vi "MainSockets.vi"() -> ()   [LabVIEW 2018]
uses:
  <vilib>/addons/zeromq/zmq_context.lvclass
  socket REP/socket REP.lvclass
  C:/Users/Denis/Desktop/communication-manager/communication-manager/Socket/Socket.lvclass
  socket REQ/socket REQ.lvclass
  socket SUB/socket SUB.lvclass
  socket PUB/socket PUB.lvclass
  RxTx/CM_RxTx.lvclass
  Socket/Socket.lvclass
panel:
  in  "socket PUB.lvclass":refnum<class "socket PUB.lvclass">
  in  "socket SUB.lvclass":refnum<class "socket SUB.lvclass">
  in  "socket REQ.lvclass":refnum<class "socket REQ.lvclass">
  in  "socket REP.lvclass":refnum<class "socket REP.lvclass">
  out "context":refnum<class "zmq_context.lvclass">
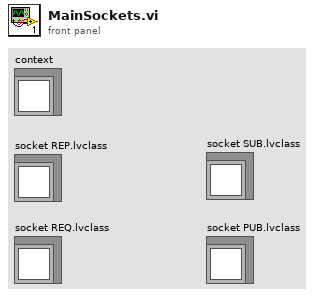
[diagram p1: front panel]
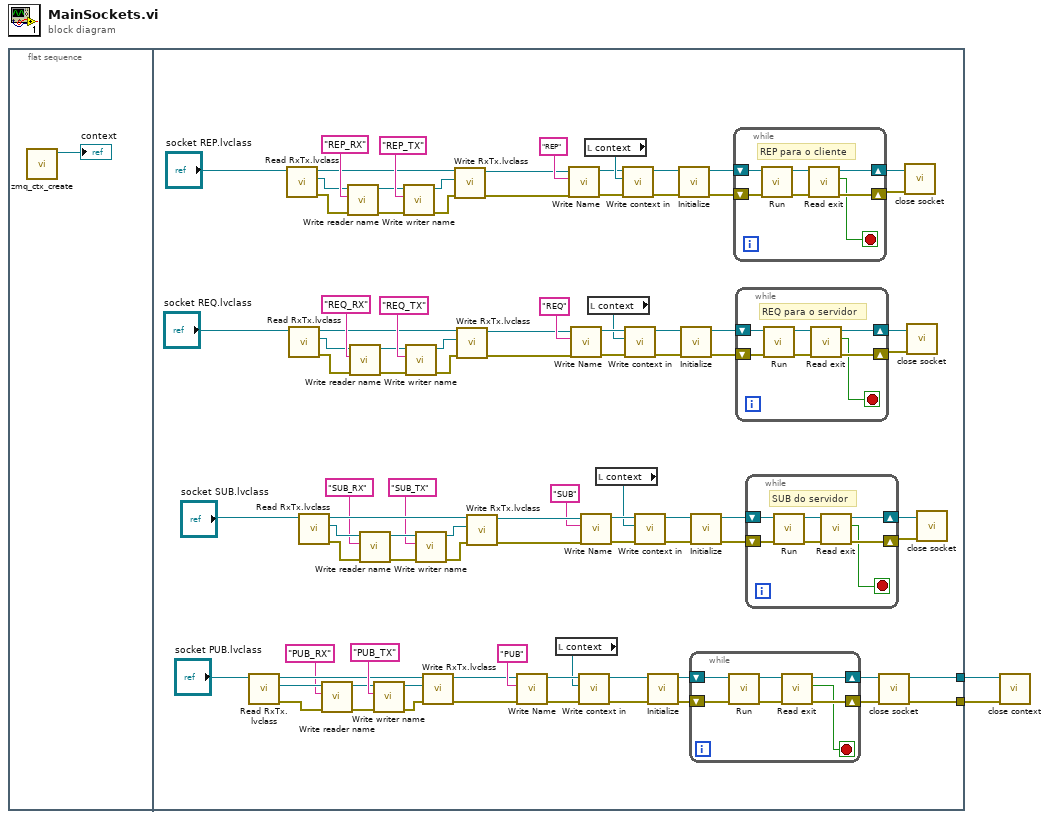
[diagram p0: block diagram]
diagram:
  n1 = flat-sequence {
    tunnel: [w7] -> w2
    tunnel: [w6] -> w1
    frame #0 {
      n2 = call <vilib>:"zmq_ctx_create.vi"() -> ("context out"=→"context":refnum<class "zmq_context.lvclass">)  [unwired: 4 in, 1 out]
    }
    frame #1 {
      n3 = call-dynamic "Read RxTx.lvclass.vi"("Socket in"="socket PUB.lvclass") -> ("error out"=w88:errorcluster, "RxTx.lvclass"=w92:refnum<class "CM_RxTx.lvclass">, "Socket out"=w89:refnum<class "socket PUB.lvclass">)  [unwired: 8 in]
      n4 = call-dynamic "Read RxTx.lvclass.vi"("Socket in"="socket REP.lvclass") -> ("error out"=w23:errorcluster, "RxTx.lvclass"=w27:refnum<class "CM_RxTx.lvclass">, "Socket out"=w24:refnum<class "socket REP.lvclass">)  [unwired: 8 in]
      n5 = call-dynamic "Read RxTx.lvclass.vi"("Socket in"="socket REQ.lvclass") -> ("error out"=w45:errorcluster, "RxTx.lvclass"=w49:refnum<class "CM_RxTx.lvclass">, "Socket out"=w46:refnum<class "socket REQ.lvclass">)  [unwired: 8 in]
      n6 = call-dynamic "Read RxTx.lvclass.vi"("Socket in"="socket SUB.lvclass") -> ("error out"=w62:errorcluster, "RxTx.lvclass"=w58:refnum<class "CM_RxTx.lvclass">, "Socket out"=w61:refnum<class "socket SUB.lvclass">)  [unwired: 8 in]
      n7 = call-dynamic "Write reader name.vi"("error in (no error)"=w88, "RX name"="PUB_RX" ("reader name"), "RxTx in"=w92) -> ("error out"=w87:errorcluster, "RxTx out"=w91:refnum<class "CM_RxTx.lvclass">)  [unwired: 7 in]
      n8 = call-dynamic "Write reader name.vi"("error in (no error)"=w23, "RX name"="REP_RX" ("reader name"), "RxTx in"=w27) -> ("error out"=w22:errorcluster, "RxTx out"=w26:refnum<class "CM_RxTx.lvclass">)  [unwired: 7 in]
      n9 = call-dynamic "Write reader name.vi"("error in (no error)"=w45, "RX name"="REQ_RX" ("reader name"), "RxTx in"=w49) -> ("error out"=w44:errorcluster, "RxTx out"=w48:refnum<class "CM_RxTx.lvclass">)  [unwired: 7 in]
      n10 = call-dynamic "Write reader name.vi"("error in (no error)"=w62, "RX name"="SUB_RX" ("reader name"), "RxTx in"=w58) -> ("error out"=w63:errorcluster, "RxTx out"=w59:refnum<class "CM_RxTx.lvclass">)  [unwired: 7 in]
      n11 = call-dynamic "Write writer name.vi"("error in (no error)"=w87, "Tx name"="PUB_TX" ("writer name"), "RxTx in"=w91) -> ("error out"=w86:errorcluster, "RxTx out"=w90:refnum<class "CM_RxTx.lvclass">)  [unwired: 7 in]
      n12 = call-dynamic "Write writer name.vi"("error in (no error)"=w22, "Tx name"="REP_TX" ("writer name"), "RxTx in"=w26) -> ("error out"=w21:errorcluster, "RxTx out"=w25:refnum<class "CM_RxTx.lvclass">)  [unwired: 7 in]
      n13 = call-dynamic "Write writer name.vi"("error in (no error)"=w44, "Tx name"="REQ_TX" ("writer name"), "RxTx in"=w48) -> ("error out"=w43:errorcluster, "RxTx out"=w47:refnum<class "CM_RxTx.lvclass">)  [unwired: 7 in]
      n14 = call-dynamic "Write writer name.vi"("error in (no error)"=w63, "Tx name"="SUB_TX" ("writer name"), "RxTx in"=w59) -> ("error out"=w64:errorcluster, "RxTx out"=w60:refnum<class "CM_RxTx.lvclass">)  [unwired: 7 in]
      n15 = call-dynamic "Write RxTx.lvclass.vi"("error in (no error)"=w86, "RxTx.lvclass"=w90, "Socket in"=w89) -> ("error out"=w4:errorcluster, "Socket out"=w5:refnum<class "socket PUB.lvclass">)  [unwired: 7 in]
      n16 = call-dynamic "Write RxTx.lvclass.vi"("error in (no error)"=w21, "RxTx.lvclass"=w25, "Socket in"=w24) -> ("error out"=w14:errorcluster, "Socket out"=w17:refnum<class "socket REP.lvclass">)  [unwired: 7 in]
      n17 = call-dynamic "Write RxTx.lvclass.vi"("error in (no error)"=w43, "RxTx.lvclass"=w47, "Socket in"=w46) -> ("error out"=w38:errorcluster, "Socket out"=w41:refnum<class "socket REQ.lvclass">)  [unwired: 7 in]
      n18 = call-dynamic "Write RxTx.lvclass.vi"("error in (no error)"=w64, "RxTx.lvclass"=w60, "Socket in"=w61) -> ("error out"=w69:errorcluster, "Socket out"=w66:refnum<class "socket SUB.lvclass">)  [unwired: 7 in]
      n19 = call-dynamic "Write Name.vi"("error in (no error)"=w4, "Name"="PUB", "Socket in"=w5) -> ("error out"=w83:errorcluster, "Socket out"=w85:refnum<class "socket PUB.lvclass">)  [unwired: 7 in]
      n20 = local read "context"() -> (w76:refnum<class "zmq_context.lvclass">)
      n21 = call-dynamic "Write Name.vi"("error in (no error)"=w14, "Name"="REP", "Socket in"=w17) -> ("error out"=w13:errorcluster, "Socket out"=w16:refnum<class "socket REP.lvclass">)  [unwired: 7 in]
      n22 = call-dynamic "Write Name.vi"("error in (no error)"=w38, "Name"="REQ", "Socket in"=w41) -> ("error out"=w37:errorcluster, "Socket out"=w40:refnum<class "socket REQ.lvclass">)  [unwired: 7 in]
      n23 = call-dynamic "Write context in.vi"("error in (no error)"=w83, "zeromq.lvlib:ZeroMQ Context"=w76, "Socket in"=w85) -> ("error out"=w82:errorcluster, "Socket out"=w84:refnum<class "socket PUB.lvclass">)  [unwired: 7 in]
      n24 = call-dynamic "Write Name.vi"("error in (no error)"=w69, "Name"="SUB", "Socket in"=w66) -> ("error out"=w70:errorcluster, "Socket out"=w67:refnum<class "socket SUB.lvclass">)  [unwired: 7 in]
      n25 = local read "context"() -> (w18:refnum<class "zmq_context.lvclass">)
      n26 = local read "context"() -> (w30:refnum<class "zmq_context.lvclass">)
      n27 = local read "context"() -> (w55:refnum<class "zmq_context.lvclass">)
      n28 = call-dynamic "Write context in.vi"("error in (no error)"=w13, "zeromq.lvlib:ZeroMQ Context"=w18, "Socket in"=w16) -> ("error out"=w12:errorcluster, "Socket out"=w15:refnum<class "socket REP.lvclass">)  [unwired: 7 in]
      n29 = call-dynamic "Write context in.vi"("error in (no error)"=w37, "zeromq.lvlib:ZeroMQ Context"=w30, "Socket in"=w40) -> ("error out"=w36:errorcluster, "Socket out"=w39:refnum<class "socket REQ.lvclass">)  [unwired: 7 in]
      n30 = call-dynamic "Write context in.vi"("error in (no error)"=w70, "zeromq.lvlib:ZeroMQ Context"=w55, "Socket in"=w67) -> ("error out"=w71:errorcluster, "Socket out"=w68:refnum<class "socket SUB.lvclass">)  [unwired: 7 in]
      n31 = call-dynamic "Initialize.vi"("error in (no error)"=w82, "socket PUB in"=w84) -> ("error out"=w79:errorcluster, "socket PUB out"=w81:refnum<class "socket PUB.lvclass">)  [unwired: 8 in]
      n32 = call-dynamic "Initialize.vi"("error in (no error)"=w12, "socket REP in"=w15) -> ("error out"=w9:errorcluster, "socket REP out"=w11:refnum<class "socket REP.lvclass">)  [unwired: 8 in]
      n33 = call-dynamic "Initialize.vi"("error in (no error)"=w36, "socket REQ in"=w39) -> ("error out"=w33:errorcluster, "socket REQ out"=w35:refnum<class "socket REQ.lvclass">)  [unwired: 8 in]
      n34 = while {
        shift-right: [w117] -> w80
        shift-left: w81 -> [w121]
        shift-right: [w116] -> w78
        shift-left: w79 -> [w120]
        stop <- w115 stop-if-true
        n35 = call-dynamic "Run.vi"("error in (no error)"=w120, "socket PUB in"=w121) -> ("error out"=w119:errorcluster, "socket PUB out"=w118:refnum<class "socket PUB.lvclass">)  [unwired: 8 in]
        n36 = call-dynamic "Read exit.vi"("error in (no error)"=w119, "Socket in"=w118) -> ("error out"=w116:errorcluster, "exit"=w115:bool, "Socket out"=w117:refnum<class "socket PUB.lvclass">)  [unwired: 7 in]
      }
      n37 = call-dynamic "Initialize.vi"("error in (no error)"=w71, "socket SUB in"=w68) -> ("error out"=w74:errorcluster, "socket SUB out"=w72:refnum<class "socket SUB.lvclass">)  [unwired: 8 in]
      n38 = while {
        shift-right: [w98] -> w10
        shift-left: w11 -> [w100]
        shift-right: [w95] -> w8
        shift-left: w9 -> [w97]
        stop <- w94 stop-if-true
        # "REP para o cliente"
        n39 = call-dynamic "Run.vi"("error in (no error)"=w97, "socket REP in"=w100) -> ("error out"=w96:errorcluster, "socket REP out"=w99:refnum<class "socket REP.lvclass">)  [unwired: 8 in]
        n40 = call-dynamic "Read exit.vi"("error in (no error)"=w96, "Socket in"=w99) -> ("error out"=w95:errorcluster, "exit"=w94:bool, "Socket out"=w98:refnum<class "socket REP.lvclass">)  [unwired: 7 in]
      }
      n41 = while {
        shift-right: [w105] -> w34
        shift-left: w35 -> [w107]
        shift-right: [w102] -> w32
        shift-left: w33 -> [w104]
        stop <- w101 stop-if-true
        # "REQ para o servidor"
        n42 = call-dynamic "Run.vi"("error in (no error)"=w104, "socket REQ in"=w107) -> ("error out"=w103:errorcluster, "socket REQ out"=w106:refnum<class "socket REQ.lvclass">)  [unwired: 8 in]
        n43 = call-dynamic "Read exit.vi"("error in (no error)"=w103, "Socket in"=w106) -> ("error out"=w102:errorcluster, "exit"=w101:bool, "Socket out"=w105:refnum<class "socket REQ.lvclass">)  [unwired: 7 in]
      }
      n44 = while {
        shift-right: [w112] -> w73
        shift-left: w72 -> [w114]
        shift-right: [w109] -> w75
        shift-left: w74 -> [w111]
        stop <- w108 stop-if-true
        # "SUB do servidor"
        n45 = call-dynamic "Run.vi"("error in (no error)"=w111, "socket SUB in"=w114) -> ("error out"=w110:errorcluster, "socket SUB out"=w113:refnum<class "socket SUB.lvclass">)  [unwired: 8 in]
        n46 = call-dynamic "Read exit.vi"("error in (no error)"=w110, "Socket in"=w113) -> ("error out"=w109:errorcluster, "exit"=w108:bool, "Socket out"=w112:refnum<class "socket SUB.lvclass">)  [unwired: 7 in]
      }
      n47 = call "close socket.vi"("error in (no error)"=w78, "Socket in"=w80) -> ("error out"=w7:errorcluster, "Socket out"=w6:refnum<class "socket PUB.lvclass">)  [unwired: 8 in]
      n48 = call "close socket.vi"("error in (no error)"=w8, "Socket in"=w10) -> ()  [unwired: 8 in, 2 out]
      n49 = call "close socket.vi"("error in (no error)"=w32, "Socket in"=w34) -> ()  [unwired: 8 in, 2 out]
      n50 = call "close socket.vi"("error in (no error)"=w75, "Socket in"=w73) -> ()  [unwired: 8 in, 2 out]
    }
  }
  n51 = call-dynamic "close context.vi"("error in (no error)"=w2, "Socket in"=w1) -> ()  [unwired: 8 in, 2 out]
